vi "runUI.vi"(8 "error in (no error)":errorcluster, 10 "Embedded VI":string, 11 "UI in":refnum<class "UI.lvclass">) -> (0 "error out":errorcluster, 3 "UI out":refnum<class "UI.lvclass">)   [LabVIEW 2019, in "UI.lvclass"]
doc: "Once you opened the session for the UI, you want to start Running the Embedded VIs in the SubPanel. This VI plays this role. You are required to provide the Embedded VI your going to launch. In case you are using several Embedded VIs, you should pass the first one to be launched."
uses:
  UI.lvclass
  PanelFactory/PanelFactory.lvclass
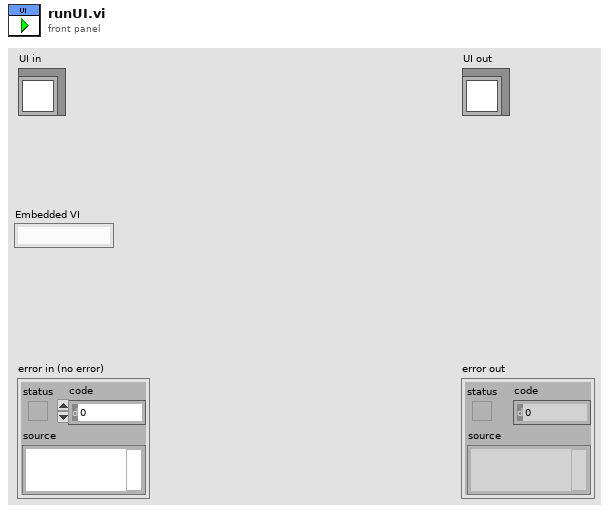
[diagram p1: front panel]
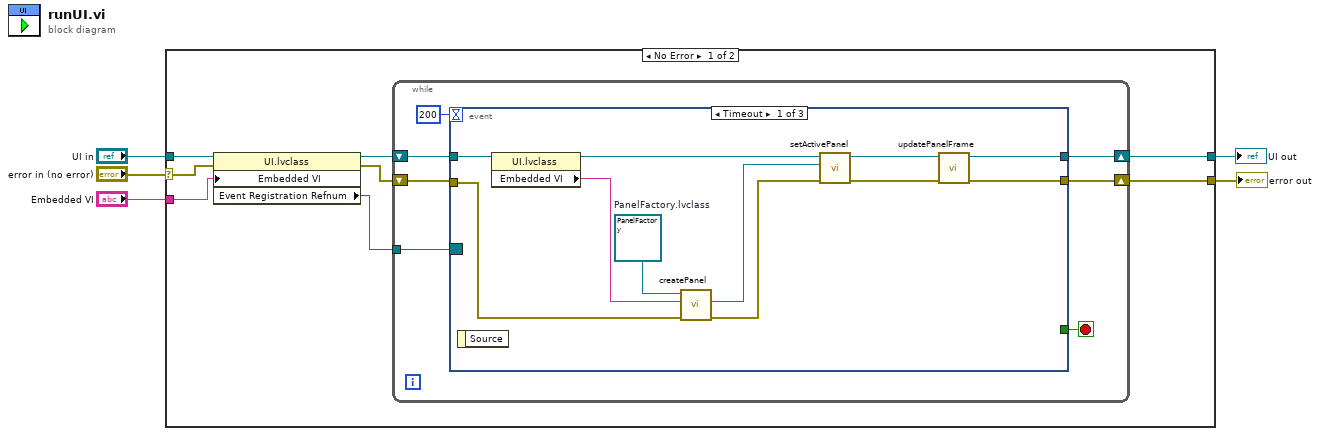
[diagram p0: block diagram]
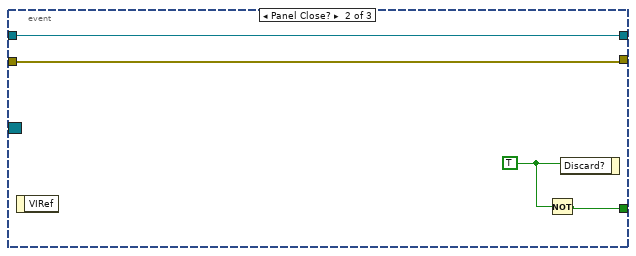
[diagram p2: hidden frame]
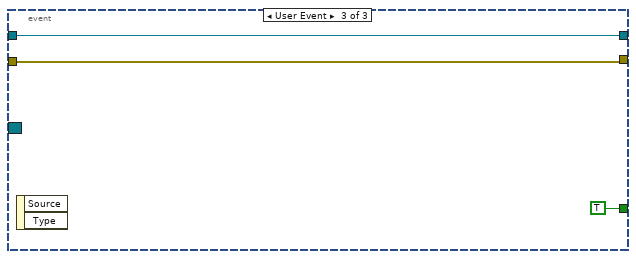
[diagram p3: hidden frame]
diagram:
  n1 = case shown="No Error" "error in (no error)" {
    selector: "error in (no error)" -> [w8 w40]
    tunnel: [w7 w40] -> w4
    tunnel: [w10 w39] -> w2
    tunnel: "UI in" -> [w9 w39]
    tunnel: "Embedded VI" -> [w6 _]
    frame No Error {
      n2 = property class="UI.lvclass"(reference=w9, error in=w8, "Embedded VI"=w6) -> (reference out=w12:refnum<class "UI.lvclass">, error out=w13:errorcluster, "Event Registration Refnum"=w11:refnum<event-registration>)
      n3 = while {
        shift-right: [w15] -> w10
        shift-left: w12 -> [w18]
        shift-right: [w14] -> w7
        shift-left: w13 -> [w19]
        tunnel: w11 -> [w16]
        stop <- w20 stop-if-true
        n4 = event shown="[0] Timeout" {
          selector: w16 -> [_ _ _]
          dyn-events: _ -> [_ _ _]
          timeout: 200 -> [_ _ _]
          tunnel: w18 -> [w31 w34 w38]
          tunnel: w19 -> [w24 w35 w37]
          tunnel: [_ w32 TRUE] -> w20
          tunnel: [w21 w34 w38] -> w15
          tunnel: [w23 w35 w37] -> w14
          event Timeout {
            w29 = refnum<class "PanelFactory.lvclass"> refnum  # PanelFactory.lvclass
            n5 = event-data() -> ()  [unwired: 1 in, 1 out]
            n6 = property class="UI.lvclass"(reference=w31) -> (reference out=w27:refnum<class "UI.lvclass">, "Embedded VI"=w26:string)  [unwired: 1 in, 1 out]
            n7 = call "createPanel.vi"("error in (no error)"=w24, "Path"=w26, "PanelFactory in"=w29) -> ("error out"=w25:errorcluster, "Panel out"=w28:refnum<class "Panel.lvclass">)  [unwired: 7 in]
            n8 = call "setActivePanel.vi"("error in (no error)"=w25, "Panel"=w28, "UI in"=w27) -> ("error out"=w30:errorcluster, "UI out"=w22:refnum<class "UI.lvclass">)  [unwired: 7 in]
            n9 = call "updatePanelFrame.vi"("error in (no error)"=w30, "UI in"=w22) -> ("error out"=w23:errorcluster, "UI out"=w21:refnum<class "UI.lvclass">)  [unwired: 8 in]
          }
          event Panel Close? {
            w33 = TRUE
            n10 = event-data() -> ()  [unwired: 1 in, 1 out]
            n11 = Not(x=w33) -> (.not. x?=w32:bool)
            n12 = event-data("Discard?"=w33) -> ()  [unwired: 1 in, 1 out]
          }
          event User Event {
            n13 = event-data() -> ()  [unwired: 1 in, 2 out]
          }
        }
      }
    }
    frame Error {
    }
  }
  "error out" <- w4
  "UI out" <- w2
